vi "Shall I start.vi"(8 "error in (no error)":errorcluster, 11 "Guardian in":refnum<class "Guardian.lvclass">) -> (0 "error out":errorcluster, 3 "Guardian out":refnum<class "Guardian.lvclass">)   [LabVIEW 2026, in "TALOS.lvlib" / "Guardian.lvlib" / "Guardian.lvclass"]
uses:
  Guardian.lvclass
  C:/LabVIEW Code/TALOS/talos/Ancestor/Ancestor/Ancestor.lvclass
  Ancestor/Ancestor/Ancestor.lvclass/Ancestor.ctl
  ea031457-16d6-41f6-b30e-12ca594b4f1c.vi
  Support VIs/Global Constants.vi
  <vilib>/Comparison/Equal/Equal Functor/Equal Functor.lvclass
  TALOS.lvlib
  Ancestor/Ancestor/Ancestor.lvclass
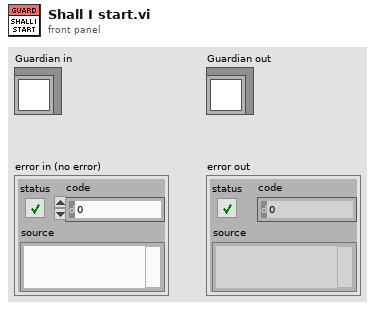
[diagram p1: front panel]
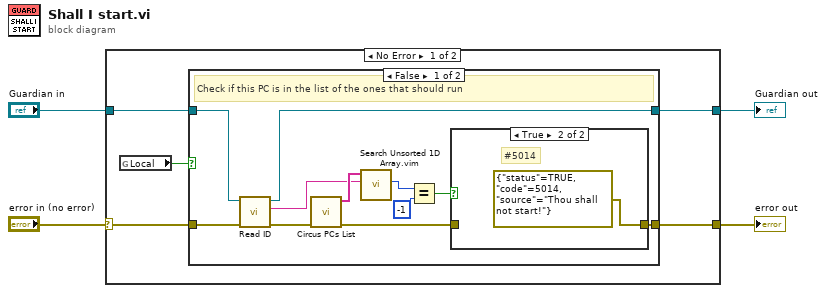
[diagram p0: block diagram]
diagram:
  n1 = case shown="No Error" "error in (no error)" {
    selector: "error in (no error)" -> [w7 w25]
    tunnel: "Guardian in" -> [w9 w26]
    tunnel: [w8 w26] -> w3
    tunnel: [w6 w25] -> w1
    frame No Error {
      n2 = global read "Global Constants.vi" "Local"() -> (w5:bool)
      n3 = case shown="False" w5 {
        tunnel: w9 -> [w20 w24]
        tunnel: [w19 w24] -> w8
        tunnel: w7 -> [w18 w23]
        tunnel: [w10 w23] -> w6
        frame False {
          # "Check if this PC is in the list of the ones that should run"
          n4 = call "Read ID.vi"("error in (no error)"=w18, "Ancestor in"=w20) -> ("error out"=w17:errorcluster, "ID"=w15:string, "Ancestor out"=w19:refnum<class "Guardian.lvclass">)  [unwired: 7 in]
          n5 = call "Circus PCs List.vi"("error in (no error)"=w17) -> ("error out"=w11:errorcluster, "PC List out"=w16:string[])  [unwired: 9 in]
          n6 = call "Search Unsorted 1D Array.vim"("element"=w15, "unsorted 1D array"=w16) -> ("index of element"=w14:i32)  [unwired: 9 in]
          n7 = Equal?(x=w14, y=-1) -> (x = y?=w12:bool)
          n8 = case shown="True" w12 {
            tunnel: w11 -> [w21 _]
            tunnel: [w21 errorcluster {"status"=TRUE, "code"=5014, "source"="Thou shall not start!"} ("error out")] -> w10
            frame False {
            }
            frame True {
              # "#5014"
            }
          }
        }
        frame True {
          # "It's in locale, just boot normally."
        }
      }
    }
    frame Error {
    }
  }
  "Guardian out" <- w3
  "error out" <- w1
